vi "create_LS370_Data_header_units.vi"() -> (3 "String":string)   [LabVIEW 2018]
uses:
  Instrument_Setup.vi
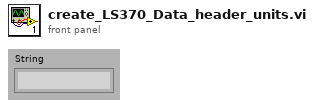
[diagram p1: front panel]
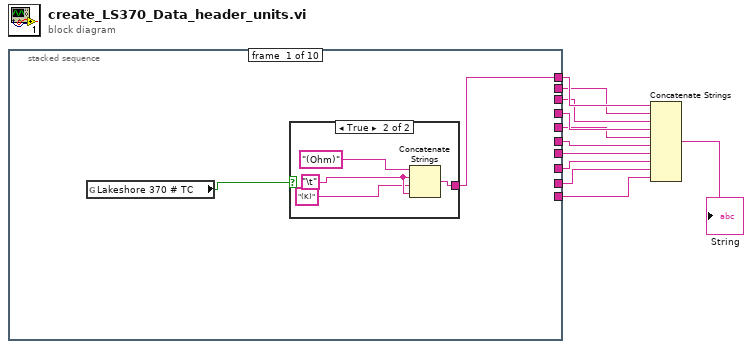
[diagram p0: block diagram]
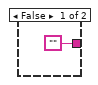
[diagram p2: hidden frame]
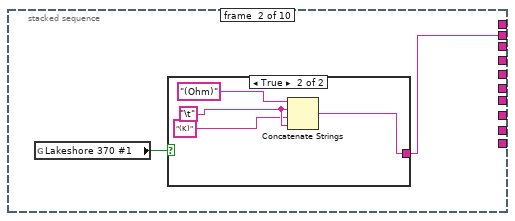
[diagram p3: hidden frame]
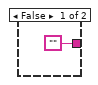
[diagram p4: hidden frame]
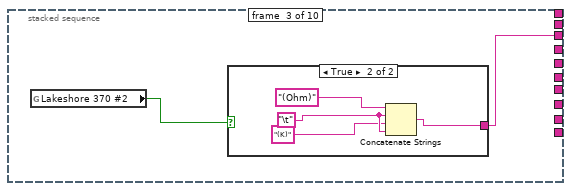
[diagram p5: hidden frame]
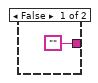
[diagram p6: hidden frame]
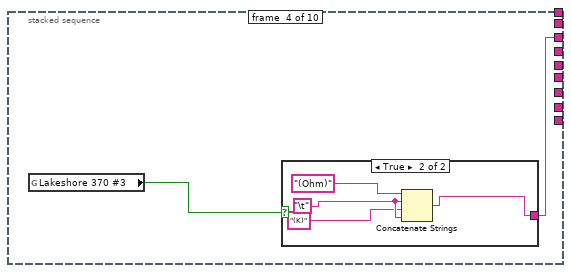
[diagram p7: hidden frame]
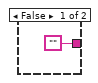
[diagram p8: hidden frame]
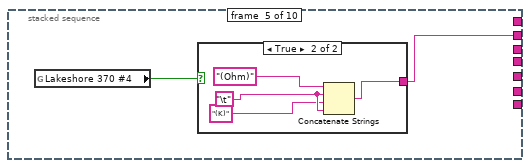
[diagram p9: hidden frame]
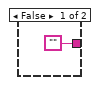
[diagram p10: hidden frame]
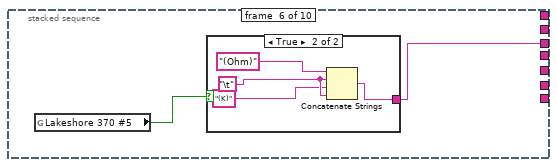
[diagram p11: hidden frame]
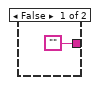
[diagram p12: hidden frame]
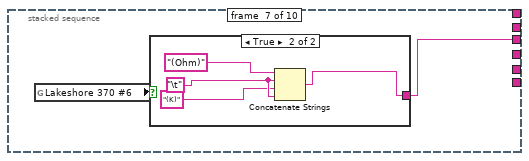
[diagram p13: hidden frame]
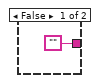
[diagram p14: hidden frame]
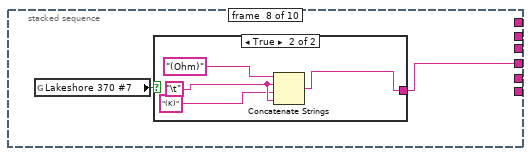
[diagram p15: hidden frame]
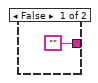
[diagram p16: hidden frame]
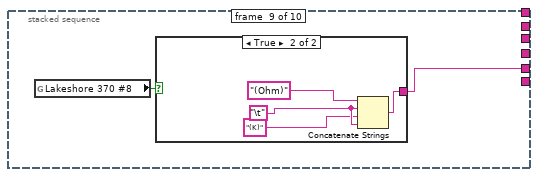
[diagram p17: hidden frame]
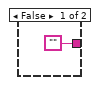
[diagram p18: hidden frame]
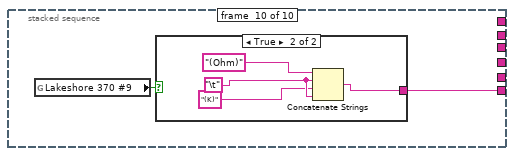
[diagram p19: hidden frame]
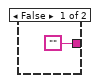
[diagram p20: hidden frame]
diagram:
  n1 = stacked-sequence {
    tunnel: [w12 _ _ _ _ _ _ _ _ _] -> w11
    tunnel: [_ w19 _ _ _ _ _ _ _ _] -> w10
    tunnel: [_ _ w26 _ _ _ _ _ _ _] -> w9
    tunnel: [_ _ _ w33 _ _ _ _ _ _] -> w8
    tunnel: [_ _ _ _ w40 _ _ _ _ _] -> w7
    tunnel: [_ _ _ _ _ w47 _ _ _ _] -> w6
    tunnel: [_ _ _ _ _ _ w54 _ _ _] -> w5
    tunnel: [_ _ _ _ _ _ _ w61 _ _] -> w4
    tunnel: [_ _ _ _ _ _ _ _ w68 _] -> w3
    tunnel: [_ _ _ _ _ _ _ _ _ w75] -> w2
    frame #0 {
      n2 = global read "Instrument_Setup.vi" "Lakeshore 370 # TC"() -> (w13:bool)
      n3 = case shown="True" w13 {
        tunnel: ["" w18] -> w12
        frame False {
        }
        frame True {
          w16 = "\t"
          n4 = Concatenate Strings("(Ohm)", w16, "(K)", w16) -> (w18:string)
        }
      }
    }
    frame #1 {
      n5 = global read "Instrument_Setup.vi" "Lakeshore 370 #1"() -> (w20:bool)
      n6 = case shown="True" w20 {
        tunnel: ["" w22] -> w19
        frame False {
        }
        frame True {
          w24 = "\t"
          n7 = Concatenate Strings("(Ohm)", w24, "(K)", w24) -> (w22:string)
        }
      }
    }
    frame #2 {
      n8 = global read "Instrument_Setup.vi" "Lakeshore 370 #2"() -> (w27:bool)
      n9 = case shown="True" w27 {
        tunnel: ["" w29] -> w26
        frame False {
        }
        frame True {
          w31 = "\t"
          n10 = Concatenate Strings("(Ohm)", w31, "(K)", w31) -> (w29:string)
        }
      }
    }
    frame #3 {
      n11 = global read "Instrument_Setup.vi" "Lakeshore 370 #3"() -> (w34:bool)
      n12 = case shown="True" w34 {
        tunnel: ["" w36] -> w33
        frame False {
        }
        frame True {
          w38 = "\t"
          n13 = Concatenate Strings("(Ohm)", w38, "(K)", w38) -> (w36:string)
        }
      }
    }
    frame #4 {
      n14 = global read "Instrument_Setup.vi" "Lakeshore 370 #4"() -> (w41:bool)
      n15 = case shown="True" w41 {
        tunnel: ["" w43] -> w40
        frame False {
        }
        frame True {
          w45 = "\t"
          n16 = Concatenate Strings("(Ohm)", w45, "(K)", w45) -> (w43:string)
        }
      }
    }
    frame #5 {
      n17 = global read "Instrument_Setup.vi" "Lakeshore 370 #5"() -> (w48:bool)
      n18 = case shown="True" w48 {
        tunnel: ["" w50] -> w47
        frame False {
        }
        frame True {
          w52 = "\t"
          n19 = Concatenate Strings("(Ohm)", w52, "(K)", w52) -> (w50:string)
        }
      }
    }
    frame #6 {
      n20 = global read "Instrument_Setup.vi" "Lakeshore 370 #6"() -> (w55:bool)
      n21 = case shown="True" w55 {
        tunnel: ["" w57] -> w54
        frame False {
        }
        frame True {
          w59 = "\t"
          n22 = Concatenate Strings("(Ohm)", w59, "(K)", w59) -> (w57:string)
        }
      }
    }
    frame #7 {
      n23 = global read "Instrument_Setup.vi" "Lakeshore 370 #7"() -> (w62:bool)
      n24 = case shown="True" w62 {
        tunnel: ["" w64] -> w61
        frame False {
        }
        frame True {
          w66 = "\t"
          n25 = Concatenate Strings("(Ohm)", w66, "(K)", w66) -> (w64:string)
        }
      }
    }
    frame #8 {
      n26 = global read "Instrument_Setup.vi" "Lakeshore 370 #8"() -> (w69:bool)
      n27 = case shown="True" w69 {
        tunnel: ["" w71] -> w68
        frame False {
        }
        frame True {
          w73 = "\t"
          n28 = Concatenate Strings("(Ohm)", w73, "(K)", w73) -> (w71:string)
        }
      }
    }
    frame #9 {
      n29 = global read "Instrument_Setup.vi" "Lakeshore 370 #9"() -> (w76:bool)
      n30 = case shown="True" w76 {
        tunnel: ["" w78] -> w75
        frame False {
        }
        frame True {
          w80 = "\t"
          n31 = Concatenate Strings("(Ohm)", w80, "(K)", w80) -> (w78:string)
        }
      }
    }
  }
  n32 = Concatenate Strings(w11, w10, w9, w8, w7, w6, w5, w4, w3, w2) -> (→"String":string)
